vi "select function.vi"() -> ()   [LabVIEW 2016]
panel:
  out "Square root Value":dbl
  in  "Number":dbl
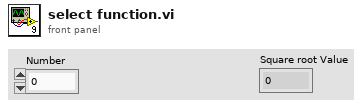
[diagram p1: front panel]
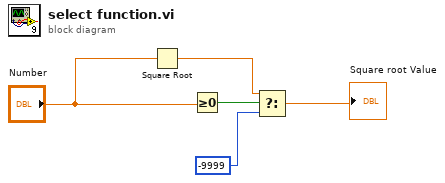
[diagram p0: block diagram]
diagram:
  n1 = Square Root(x="Number") -> (sqrt(x)=w2:dbl)
  n2 = Greater Or Equal To 0?(x="Number") -> (x >= 0?=w5:bool)
  n3 = Select(t=w2, s=w5, f=-9999) -> (s? t:f=→"Square root Value":dbl)
